vi "Test alarms and traces DSC.vi"(8 "error in (no error)":errorcluster, 11 "Experiment Name":string) -> (0 "error out":errorcluster)   [LabVIEW 2020]
uses:
  Alarms--Cluster.ctl
  Shared/MySQL/Preset Query Enum.ctl
  Alarms Info Cluster.ctl
  <vilib>/event_ctls.llb/usereventprio.ctl
  <vilib>/Utility/config.llb/Read Key (String).vi
  <vilib>/Utility/config.llb/NI_LVConfig.lvlib
panel:
  in  "Mute Alert":bool
  in  "Close":bool
  in  "Alarms Display":i32(listbox)
  out "Alarms Info":string[][](array[string])
  out "Numeric 2":i32
  out "Numeric":i32
  in  "exit":bool
  out "Process URL":string
  out "Application:Directory Path":path
  out "alarms":T1[](array[typedef])=[{"alarm URL"="\\\\LASERBAY-DEV\\Logger Master\\LB_Amp1_Energy.Alarms.LB_Amp1_Energy", "set time"=timestamp(3511959737.5175076 s since 1904-01-01), "set user"="(Nobody)", "ack time"=timestamp(-9223372036854775808 s since 1904-01-01), "ack user"="", "clear time"=timestamp(-9223372036854775808 s since 1904-01-01), "clear user"="", "setpoint"=1200.0, "value"=1409.99, "priority"=1, "alarm area"="Laser Bay", "alarm description"="LB_Amp1_Energy", "ack comment"="", "event?"=FALSE, "Refnum"=216172782113783839}] {"value" format="%.2f"; "setpoint" format="%.2f"; "clear time" format="%<%X\n%x>T"; "ack time" format="%<%X\n%x>T"; "set time" format="%<%X\n%x>T"}
  # "A\\\\LASERBAY-DEV\\Logger Master\\LB_Amp1_Energy.Alarms.LB_Amp1_EnergyÑds]Ž£p²ð‚¸(Nobody)€€@’À@—™55’ÍLaserBayHi Alarm&5\\\\LASERBAY-DEV\\Logger Master\\LB_Amp2_Energy.Alarms.LoÑ^ã“´Š˜tÖk°(Nobody)€€@9? ‡Ä9LaserBayLo Alarm7\\\\LASERBAY-DEV\\Logger Master\\LB_Energy.Alarms.LB_EnergyÑ`Þú|2€…Ð(Nobody)€€?™™™™™™š?™š¦\t¤øLaserBay\tLB_Energy"
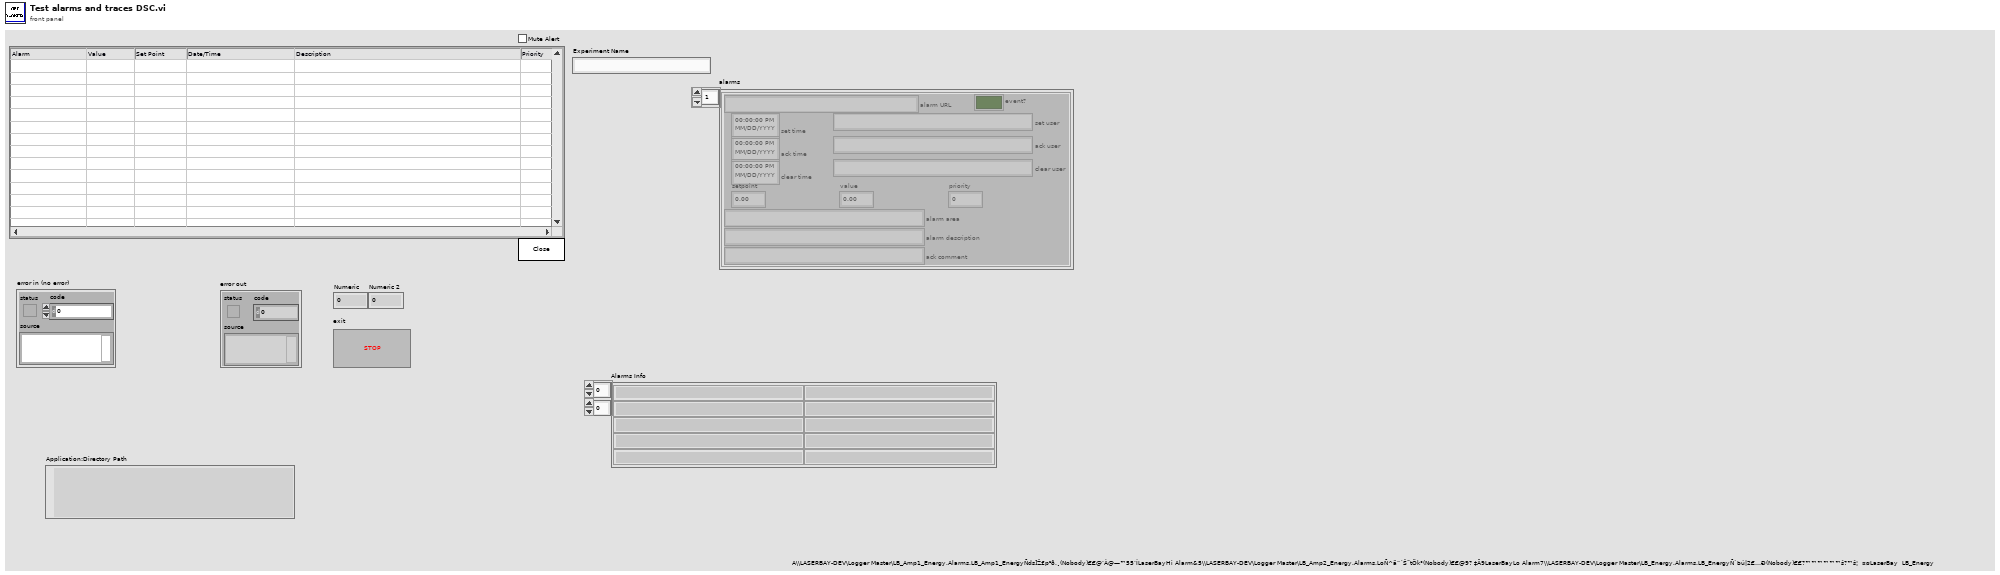
[diagram p1: front panel]
types:
  T1 = typedef "Alarms--Cluster.ctl" = cluster{"alarm URL":string, "set time":timestamp, "set user":string, "ack time":timestamp, "ack user":string, "clear time":timestamp, "clear user":string, "setpoint":dbl, "value":dbl, "priority":u32, "alarm area":string, "alarm description":string, "ack comment":string, "event?":bool, "Refnum":u64}
  T2 = typedef "Preset Query Enum.ctl" = enum16{"Get Locations", "Get all IPs and MACs", "Get classes", "Get expt variables to set at scanstart for particular device", "Get expt devices and variables with start values", "Get expt devices and variables (with data to get)", "Get expt devices with data to get", "Get Expt devices and GUIs", "Get all devices basic properties", "Get Virtual Devices Core Info", "Get Expt names", "Get experiment basic properties", "Get experiment alarm variables", "Get MC Ports", "Get device network comm port", "Get devicetype lvclass path", "Get basic device properties", "Get Init Order", "Get all setable variables of a device", "Get device variable aliases", "Get force values of all settable variables", "Get all variables of a devicetype", "Get all variables of a device", "Get plotter details", "Get Saved Scans", "Get Scan Info", "GetGeneralGUIs", "Get expt for plotter", "Get plotter IDs from expt", "Get all devices", "Get all Virtual Devices", "Get all aliases", "Get variable and device info for Virtual Device", "GetItemLocatorIP", "Get IPs for GUIs", "Get DeviceType from Device", "GetLocalPortRange", "GetDevicePresetVariables", "Get Device Configuration", "GetAllPresetNames", "GetAllConfigurationNames", "GetPresetDeviceNames"}
  T3 = typedef "NI_LVConfig.lvlib/Config Data RefNum.ctl" = refnum<k1>
  T4 = typedef "Alarms Info Cluster.ctl" = cluster{"Alarms Data":string[][], "Alert":bool, "Error":bool}
  T5 = cluster{"alarm URL":string, "set time":timestamp, "set user":string, "ack time":timestamp, "ack user":string, "clear time":timestamp, "clear user":string, "setpoint":dbl, "value":dbl, "priority":u32, "alarm area":string, "alarm description":string, "ack comment":string, "event?":bool, "Refnum":u64}[]
  T6 = enum32{"Invalid", "Standard", "Closed", "Hidden", "Minimized", "Maximized"}
  T7 = typedef "usereventprio.ctl" = enum32{"high priority", "normal priority"}
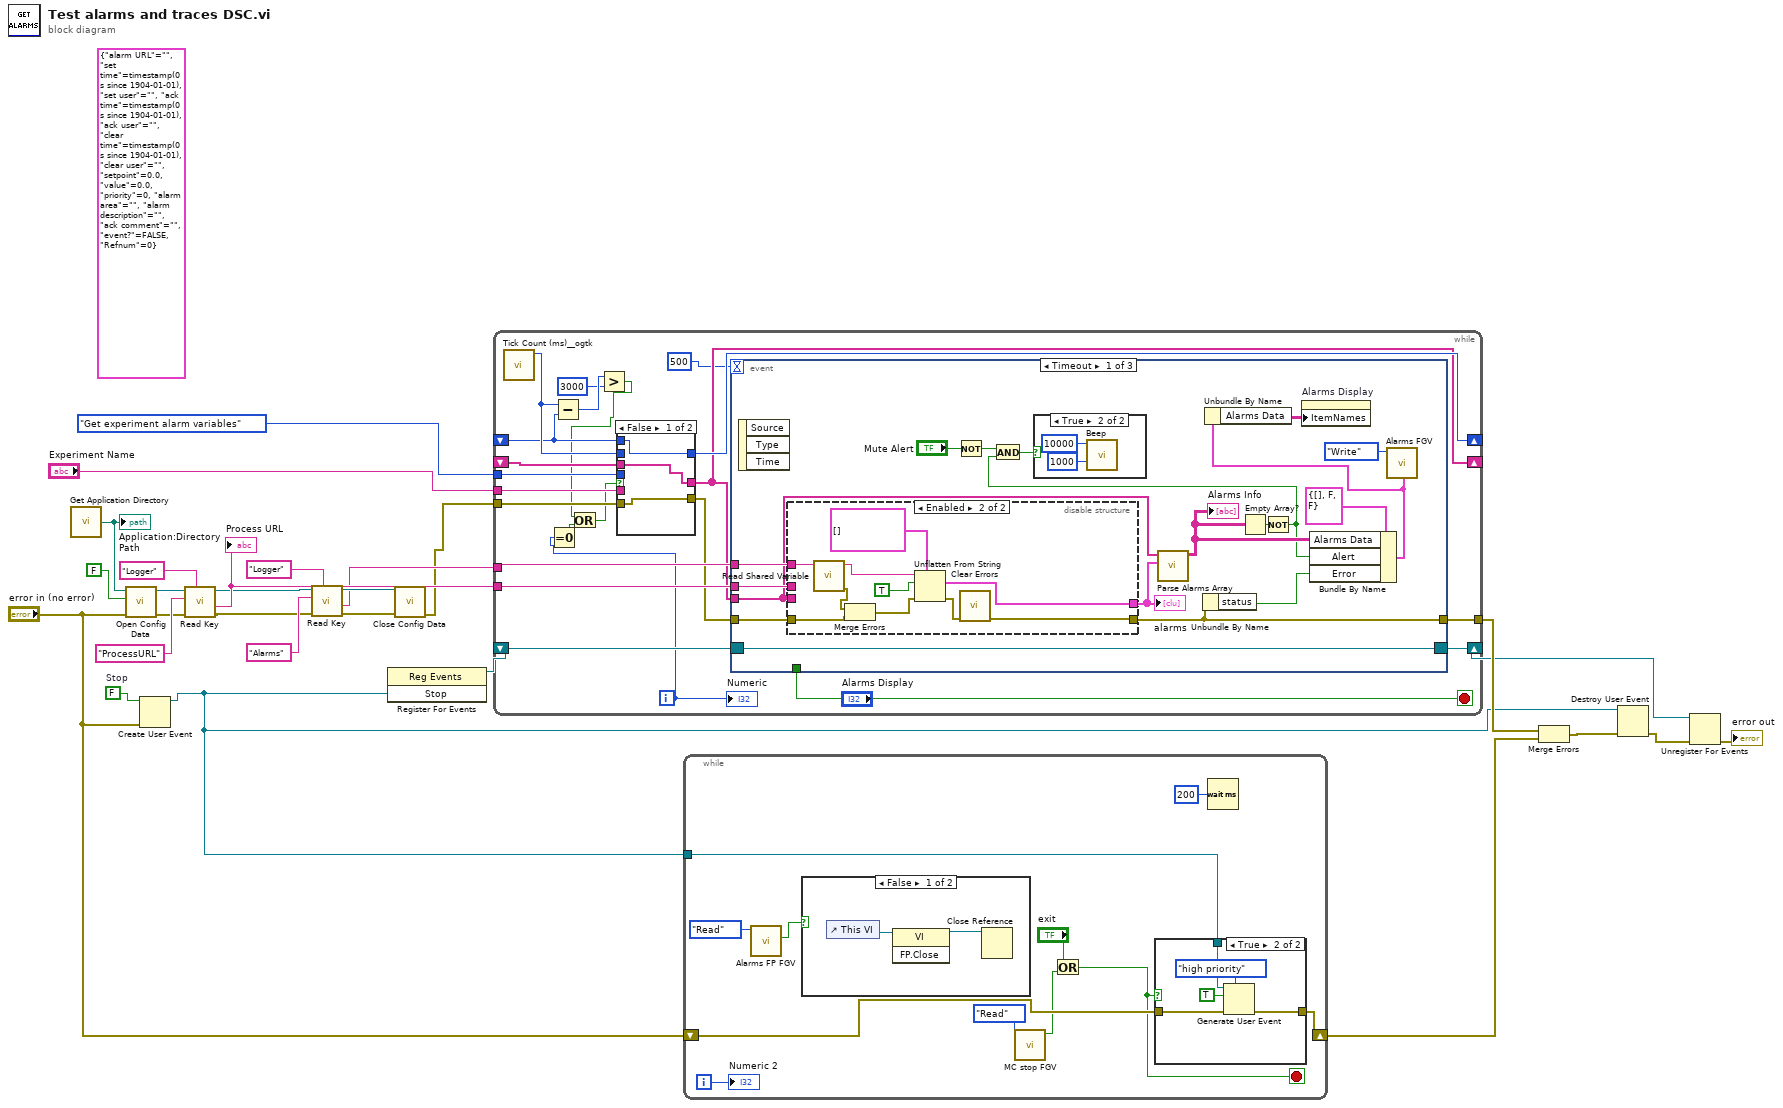
[diagram p0: block diagram]
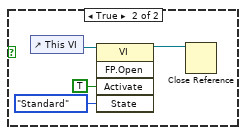
[diagram p2: hidden frame]
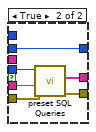
[diagram p4: hidden frame]
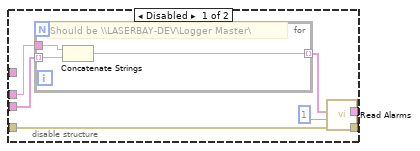
[diagram p5: hidden frame]
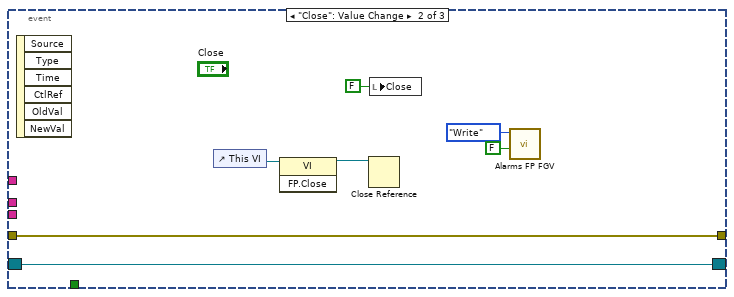
[diagram p7: hidden frame]
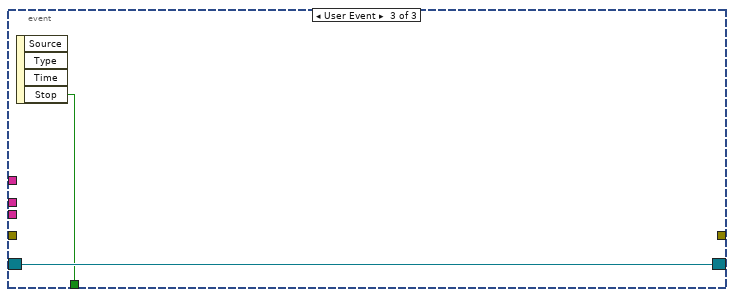
[diagram p8: hidden frame]
diagram:
  (unwired) T1 {"alarm URL"="", "set time"=timestamp(0 s since 1904-01-01), "set user"="", "ack time"=timestamp(0 s since 1904-01-01), "ack user"="", "clear time"=timestamp(0 s since 1904-01-01), "clear user"="", "setpoint"=0.0, "value"=0.0, "priority"=0, "alarm area"="", "alarm description"="", "ack comment"="", "event?"=FALSE, "Refnum"=0} ("Alarm")
  w20 = FALSE  # Stop
  n1 = call "Get Application Directory.vi"() -> ("Path to config file"=w27:path)  [unwired: 2 in]
  "Application:Directory Path" <- w27
  n2 = call <vilib>:"Open Config Data.vi"("error in (no error)"="error in (no error)", "create file if necessary (T)"=FALSE, "configuration file path"=w27) -> ("error out"=w22:errorcluster, "refnum"=w25:T3)  [unwired: 6 in, 1 out]
  n3 = Create User Event(user event datatype=w20, error in="error in (no error)") -> (user event=w11:refnum<user-event>)  [unwired: 1 out]
  n4 = call-poly <vilib>:"Read Key.vi"("section"="Logger", "error in (no error)"=w22, "key"="ProcessURL", "refnum"=w25) -> ("error out"=w6:errorcluster, "value"=w21:string, "refnum out"=w9:T3)  [unwired: 4 in, 1 out]
  "Process URL" <- w21
  n5 = call-poly <vilib>:"Read Key.vi"("section"="Logger", "error in (no error)"=w6, "key"="Alarms", "refnum"=w9) -> ("error out"=w5:errorcluster, "value"=w4:string, "refnum out"=w8:T3)  [unwired: 4 in, 1 out]
  n6 = register-events(w11) -> (reference out=w15:refnum<event-registration>)  [unwired: 2 in, 1 out]
  n7 = call <vilib>:"Close Config Data.vi"("error in (no error)"=w5, "refnum"=w8) -> ("error out"=w1:errorcluster)  [unwired: 8 in, 1 out]
  n8 = while {
    tunnel: w21 -> [w49]
    tunnel: [w47] -> w17
    shift-right: [w46] -> w12
    shift-left: w15 -> [w48]
    tunnel: w4 -> [w44]
    tunnel: Preset_Query_Enum."Get experiment alarm variables" ("Preset Query") -> [w43]
    tunnel: "Experiment Name" -> [w42]
    tunnel: w1 -> [w41]
    shift-right: [w39] -> _
    shift-left: _ -> [w34]
    shift-right: [w38] -> _
    shift-left: _ -> [w37]
    i -> [w31]
    stop <- w45 stop-if-true
    n9 = call <userlib>:"Tick Count (ms)__ogtk.vi"() -> ("millisecond timer value"=w35:u32)  [unwired: 10 in, 1 out]
    n10 = Equal To 0?(x=w31) -> (x = 0?=w30:bool)
    n11 = Subtract(x=w35, y=w34) -> (x-y=w33:u32)
    n12 = Greater?(x=w33, y=u32 3000) -> (0:w29:bool)
    n13 = Or(x=w29, y=w30) -> (x .or. y?=w28:bool)
    n14 = case shown="False" w28 {
      tunnel: w43 -> [_ w58]
      tunnel: w42 -> [_ w57]
      tunnel: [w51 w56] -> w38
      tunnel: w41 -> [w50 w55]
      tunnel: [w50 w54] -> w40
      tunnel: w35 -> [_ w53]
      tunnel: [w52 w53] -> w39
      tunnel: w34 -> [w52 _]
      tunnel: w37 -> [w51 _]
      frame False {
      }
      frame True {
        n15 = call "preset SQL Queries.vi"("error in (no error)"=w55, "Expt name / MCIP/ Variable/Preset Name"=w57, "Preset Query"=w58) -> ("error out"=w54:errorcluster, "1st column 1st data"=w56:string[])  [unwired: 6 in, 1 out]
      }
    }
    n16 = event shown="[0] Timeout" {
      selector: w48 -> [w73 w103 w107]
      dyn-events: [w73 w103 w107] -> w46
      timeout: 500 -> [_ _ _]
      tunnel: w38 -> [w59 _ _]
      tunnel: w40 -> [w76 w104 _]
      tunnel: w49 -> [w75 _ _]
      tunnel: [w70 w104 _] -> w47
      tunnel: [_ _ w106] -> w45
      tunnel: w44 -> [w63 _ _]
      event Timeout {
        n17 = event-data() -> ()  [unwired: 1 in, 3 out]
        n18 = disable-structure shown="Enabled" {
          disable-tunnel: w59 -> [w83 _]
          disable-tunnel: w76 -> [w80 w90]
          disable-tunnel: w75 -> [w79 _]
          disable-tunnel: [w78 w93] -> w72
          disable-tunnel: [w77 w94] -> w70
          disable-tunnel: w63 -> [_ w87]
          frame Disabled {
            n19 = for {
              tunnel: w83 -> [w86] mode=indexing
              tunnel: [w85] -> w81 mode=indexing
              tunnel: w79 -> [w84]
              # "Should be \\\\LASERBAY-DEV\\Logger Master\\"
              n20 = Concatenate Strings(w84, w86) -> (w85:string)
            }
            n21 = call <vilib>:"Read Alarms.vi"("error in (no error)"=w80, "timeout (s)"=1, "shared variables"=w81) -> ("error out"=w77:errorcluster, "alarms"=w78:T5)  [unwired: 7 in]
          }
          frame Enabled {
            n22 = call "Read Shared Variable.vi"("String"=w87) -> ("error out"=w88:errorcluster, "Value out"=w91:string)  [unwired: 9 in]
            n23 = Merge Errors(w88, w90) -> (w89:errorcluster)
            n24 = Unflatten From String(type=T1[] [] ("alarms 2"), binary string=w91, data includes array or string size? (T)=TRUE, error in (no error)=w89) -> (value=w93:T1[], error out=w95:errorcluster)  [unwired: 1 in, 1 out]
            n25 = call <vilib>:"Clear Errors.vi"("error in (no error)"=w95) -> ("error out"=w94:errorcluster)  [unwired: 5 in, 1 out]
          }
        }
        "alarms" <- w72
        n26 = Not(x="Mute Alert") -> (.not. x?=w64:bool)
        n27 = call "Parse Alarms Array.vi"("alarms"=w72, "Alarms for Expt"=w59) -> ("Alarms Info"=w62:string[][])  [unwired: 9 in]
        "Alarms Info" <- w62
        n28 = Unbundle By Name(w70) -> ("status"=w69:bool)
        n29 = Empty Array?(array=w62) -> (empty?=w61:bool)
        n30 = Not(x=w61) -> (.not. x?=w60:bool)
        n31 = And(x=w64, y=w60) -> (x .and. y?=w65:bool)
        n32 = case shown="True" w65 {
          frame False {
          }
          frame True {
            n33 = call <vilib>:"Beep.vi"("duration (msec)"=u32 1000, "frequency (Hz)"=u32 10000) -> ()  [unwired: 10 in]
          }
        }
        n34 = Bundle By Name(cluster=T4 {"Alarms Data"=[], "Alert"=FALSE, "Error"=FALSE} ("Alarms Info Out"), "Alarms Data"=w62, "Alert"=w60, "Error"=w69) -> (w68:T4)
        n35 = Unbundle By Name(w68) -> ("Alarms Data"=w67:string[][])
        n36 = property on="Alarms Display" class="MCListbox (strict)"("ItemNames"=w67) -> ()  [unwired: 2 in, 2 out]
        n37 = call "Alarms FGV.vi"("Alarms Info"=w68, "Function"=enum16{"Read", "Write", "Clear"}."Write") -> ()  [unwired: 5 in, 1 out]
      }
      event "Close": Value Change {
        n38 = event-data() -> ()  [unwired: 1 in, 6 out]
        n39 = control-ref of="This VI"() -> (w101:refnum<vi>)
        n40 = invoke class="VI" method="FP.Close"(reference=w101) -> (reference out=w102:refnum<vi>)  [unwired: 2 in, 2 out]
        n41 = Close Reference(reference=w102) -> ()  [unwired: 1 in, 1 out]
        n42 = local write "Close"(FALSE ("Close")) -> ()
        n43 = call "Alarms FP FGV.vi"("FP Open in"=FALSE, "Function"=enum16{"Read", "Write", "Clear"}."Write") -> ()  [unwired: 5 in, 1 out]
      }
      event User Event {
        n44 = event-data() -> ("Stop"=w106:bool)  [unwired: 1 in, 3 out]
      }
    }
    "Numeric" <- w31
  }
  n45 = while {
    tunnel: w11 -> [w116]
    shift-right: [w115] -> w18
    shift-left: "error in (no error)" -> [w114]
    i -> [w110]
    stop <- w111 stop-if-true
    n46 = call "Alarms FP FGV.vi"("Function"=enum16{"Read", "Write", "Clear"}."Read") -> ("FP Open out"=w108:bool)  [unwired: 6 in]
    n47 = case shown="False" w108 {
      frame False {
        n48 = control-ref of="This VI"() -> (w120:refnum<vi>)
        n49 = invoke class="VI" method="FP.Close"(reference=w120) -> (reference out=w119:refnum<vi>)  [unwired: 2 in, 2 out]
        n50 = Close Reference(reference=w119) -> ()  [unwired: 1 in, 1 out]
      }
      frame True {
        n51 = control-ref of="This VI"() -> (w124:refnum<vi>)
        n52 = invoke class="VI" method="FP.Open"(reference=w124, "Activate"=TRUE ("Activate?"), "State"=T6."Standard") -> (reference out=w121:refnum<vi>)  [unwired: 2 in, 4 out]
        n53 = Close Reference(reference=w121) -> ()  [unwired: 1 in, 1 out]
      }
    }
    n54 = call "MC stop FGV.vi"("Function"=enum16{"Read", "Write", "Clear"}."Read") -> ("Stop out"=w112:bool)  [unwired: 9 in, 1 out]
    n55 = Or(x="exit", y=w112) -> (x .or. y?=w111:bool)
    n56 = case shown="True" w111 {
      tunnel: w116 -> [_ w130]
      tunnel: [w125 w128] -> w115
      tunnel: w114 -> [w125 w127]
      frame False {
      }
      frame True {
        n57 = Generate User Event(priority (normal)=usereventprio."high priority", user event=w130, event data cluster=TRUE ("event data"), error in=w127) -> (error out=w128:errorcluster)  [unwired: 1 out]
      }
    }
    n58 = Wait (ms)(milliseconds to wait=u32 200) -> ()  [unwired: 1 out]
    "Numeric 2" <- w110
  }
  n59 = Merge Errors(w17, w18) -> (w14:errorcluster)
  n60 = Destroy User Event(user event=w11, error in=w14) -> (error out=w13:errorcluster)
  n61 = Unregister For Events(event registration refnum=w12, error in=w13) -> (error out=→"error out":errorcluster)
